vi "TDMSAdv deleteMultiDatas.vi"(5 "group name":string, 7 "channel names":string[](array[string]), 8 "error in (no error)":errorcluster, 9 "deleteNames":string[](array[string]), 10 "deleteIndex":i32[](array[numeric]), 11 "TDMSAdv in":refnum<class "TDMSAdv.lvclass">=refnum) -> (0 "error out":errorcluster, 3 "TDMSAdv out":refnum<class "TDMSAdv.lvclass">)   [LabVIEW 2018, in "TDMSAdv.lvclass"]
uses:
  TDMSAdv.lvclass
  TDMSAdv.lvclass/TDMSAdv.ctl
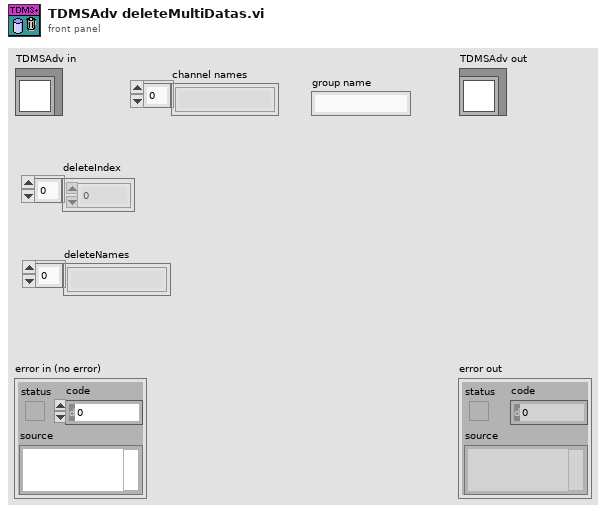
[diagram p1: front panel]
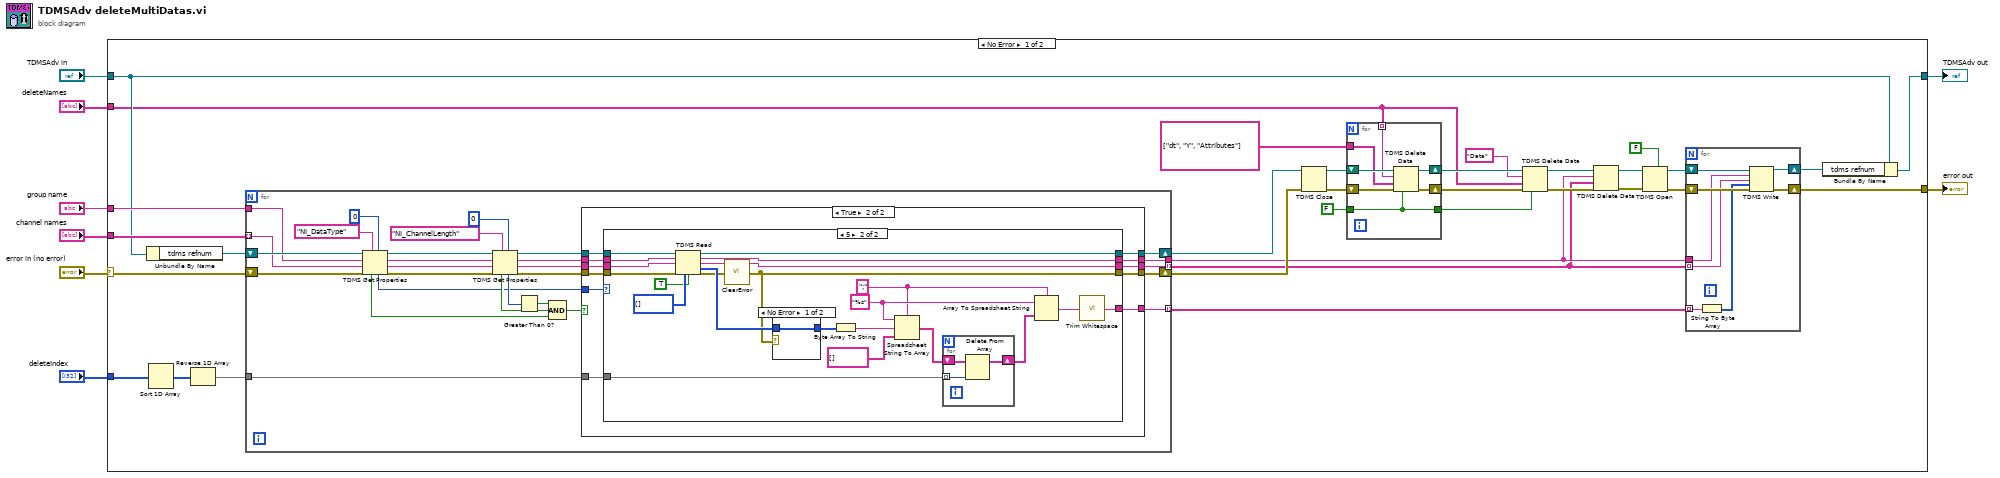
[diagram p0: block diagram]
diagram:
  n1 = case shown="No Error" "error in (no error)" {
    selector: "error in (no error)" -> [w40 w130]
    tunnel: [w18 w130] -> w7
    tunnel: [w39 w129] -> w5
    tunnel: "TDMSAdv in" -> [w20 w129]
    tunnel: "channel names" -> [w38 _]
    tunnel: "group name" -> [w29 _]
    tunnel: "deleteNames" -> [w16 _]
    tunnel: "deleteIndex" -> [w24 _]
    frame No Error {
      n2 = Unbundle By Name(w20) -> ("tdms refnum"=w35:refnum<k34>)
      n3 = Sort 1D Array(array=w24) -> (sorted array=w23:i32[])
      n4 = Reverse 1D Array(array=w23) -> (reversed array=w22:i32[])
      n5 = for {
        tunnel: w29 -> [w61]
        tunnel: w38 -> [w60] mode=indexing
        shift-right: [w63] -> w21
        shift-left: w40 -> [w65]
        shift-right: [w62] -> w26
        shift-left: w35 -> [w64]
        tunnel: [w59] -> w13
        tunnel: [w58] -> w12 mode=indexing
        tunnel: [w57] -> w25 mode=indexing
        tunnel: w22 -> [w56]
        n6 = TDMS Get Properties(5:u16 0, 7:"NI_DataType" ("property name"), 8:w65, 9:w60, 10:w61, 11:w64) -> (0:w81:errorcluster, 1:w78:string, 2:w79:string, 3:w80:refnum<k34>, 4:w66:u16, 6:w69:bool)
        n7 = TDMS Get Properties(5:u64 0, 7:"NI_ChannelLength" ("property name"), 8:w81, 9:w78, 10:w79, 11:w80) -> (0:w72:errorcluster, 1:w73:string, 2:w74:string, 3:w75:refnum<k34>, 4:w67:u64, 6:w68:bool)
        n8 = Greater Than 0?(x=w67) -> (x > 0?=w71:bool)
        n9 = Compound Arithmetic op=AND(w71, w68, w69) -> (w70:bool)
        n10 = case shown="True" w70 {
          tunnel: [w87 w91] -> w63
          tunnel: w75 -> [w86 w98]
          tunnel: w72 -> [w87 w95]
          tunnel: w74 -> [w85 w97]
          tunnel: w73 -> [w84 w96]
          tunnel: w66 -> [_ w94]
          tunnel: [_ w93] -> w57
          tunnel: [w86 w92] -> w62
          tunnel: [w85 w90] -> w59
          tunnel: [w84 w89] -> w58
          tunnel: w56 -> [_ w88]
          frame False {
          }
          frame True {
            n11 = case shown="5" w94 {
              tunnel: [w99 w122] -> w91
              tunnel: [_ w103] -> w93
              tunnel: w98 -> [w102 w116]
              tunnel: w95 -> [w99 w119]
              tunnel: w97 -> [w101 w117]
              tunnel: w96 -> [w100 w118]
              tunnel: [w102 w114] -> w92
              tunnel: [w101 w113] -> w90
              tunnel: [w100 w112] -> w89
              tunnel: w88 -> [_ w109]
              frame Default {
              }
              frame 5 {
                w107 = "%s" ("format string")
                w106 = ";"
                n12 = TDMS Read(0:w116, 5:w117, 7:w118, 11:w119, 12:u8[] [], 13:TRUE ("return channels in file order? (F)")) -> (4:w114:refnum<k34>, 6:w113:string, 8:w112:string, 10:w124:u8[], 15:w121:errorcluster)  [unwired: 2 in, 1 out]
                n13 = call <vilib>:"ClearError.vi"("error in (no error)"=w121) -> ("error out"=w122:errorcluster)
                n14 = case shown="No Error" w122 {
                  tunnel: w124 -> [w128 _]
                  tunnel: [w128 _] -> w115
                  frame No Error {
                  }
                  frame Error {
                  }
                }
                n15 = Byte Array To String(unsigned byte array=w115) -> (string=w110:string)
                n16 = Spreadsheet String To Array(delimiter (Tab)=w106, format string=w107, spreadsheet string=w110, array type (2D Dbl)=string[] []) -> (array=w108:string[])
                n17 = for {
                  tunnel: w109 -> [w127] mode=indexing
                  shift-right: [w125] -> w105
                  shift-left: w108 -> [w126]
                  n18 = Delete From Array(array=w126, index=w127) -> (array with subset deleted=w125:string[])  [unwired: 1 in, 1 out]
                }
                n19 = Array To Spreadsheet String(delimiter (Tab)=w106, array=w105, 3:w107) -> (spreadsheet string=w104:string)
                n20 = call <vilib>:"Trim Whitespace.vi"("string"=w104) -> ("trimmed string"=w103:string)  [unwired: 1 in]
              }
            }
          }
        }
      }
      n21 = TDMS Close(8:w21, 11:w26) -> (0:w36:errorcluster, 3:w37:path)
      n22 = for {
        shift-right: [w53] -> w33
        shift-left: w37 -> [w55]
        shift-right: [w52] -> w32
        shift-left: w36 -> [w54]
        tunnel: string[] ["dt", "Y", "Attributes"] ("channel name(s) in") -> [w51]
        tunnel: FALSE ("keep empty group/channel? (T)") -> [w50]
        tunnel: [w50] -> w30
        tunnel: w16 -> [w49] mode=indexing
        n23 = TDMS Delete Data(6:w50, 8:w54, 9:w51, 10:w49, 11:w55) -> (0:w52:errorcluster, 3:w53:path)  [unwired: 2 in]
      }
      n24 = TDMS Delete Data(6:w30, 8:w32, 9:w16, 10:"Data" ("group name in"), 11:w33) -> (0:w14:errorcluster, 3:w15:path)  [unwired: 2 in]
      n25 = TDMS Delete Data(8:w14, 9:w12, 10:w13, 11:w15) -> (0:w11:errorcluster, 3:w10:path)  [unwired: 3 in]
      n26 = TDMS Open(5:FALSE ("create index file? (T)"), 8:w11, 11:w10) -> (0:w27:errorcluster, 3:w28:refnum<k34>)  [unwired: 4 in]
      n27 = for {
        tunnel: w12 -> [w45] mode=indexing
        tunnel: w25 -> [w44] mode=indexing
        tunnel: w13 -> [w46]
        shift-right: [w42] -> w19
        shift-left: w28 -> [w48]
        shift-right: [w41] -> w18
        shift-left: w27 -> [w47]
        n28 = String To Byte Array(string=w44) -> (unsigned byte array=w43:u8[])
        n29 = TDMS Write(0:w48, 5:w46, 7:w45, 9:w43, 11:w47) -> (4:w42:refnum<k34>, 15:w41:errorcluster)  [unwired: 1 in, 2 out]
      }
      n30 = Bundle By Name(cluster=w20, "tdms refnum"=w19) -> (w39:refnum<class "TDMSAdv.lvclass">)
    }
    frame Error {
    }
  }
  "error out" <- w7
  "TDMSAdv out" <- w5
